vi "实时小时数据处理整合 (子VI).vi"(11 "枚举":enum16{"实时数据排序", "小时数据排序"}(ring)) -> (3 "已排序的数组":string[](array[string]))   [LabVIEW 2016, in "数据传输系统.lvlib"]
uses:
  <userlib>/_OpenG.lib/array/array.llb/Remove Duplicates from 1D Array (String)__ogtk.vi
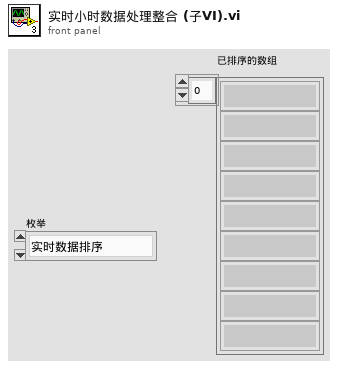
[diagram p1: front panel]
types:
  T1 = cluster{"PH":string[][], "CODCr":string[][], "氨氮":string[][], "CODMn":string[][], "总氮":string[][], "总磷":string[][], "电导率":string[][], "水温":string[][], "DO":string[][], "浊度":string[][], "叶绿素":string[][], "藻密度":string[][], "铜":string[][], "盐度":string[][], "水位":string[][], "流速":string[][], "瞬时流量":string[][], "累积流量":string[][], "亚硝酸盐":string[][], "硫化物":string[][], "ORP":string[][], "铅":string[][], "镉":string[][], "锌":string[][], "镍":string[][], "锰":string[][], "汞":string[][], "气温":string[][], "气压":string[][], "风速":string[][], "风向":string[][], "盐度 2":string[][], "磷酸盐":string[][], "硝氮":string[][], "氟化物":string[][], "挥发酚":string[][], "氯化物":string[][], "蓝绿藻":string[][]}
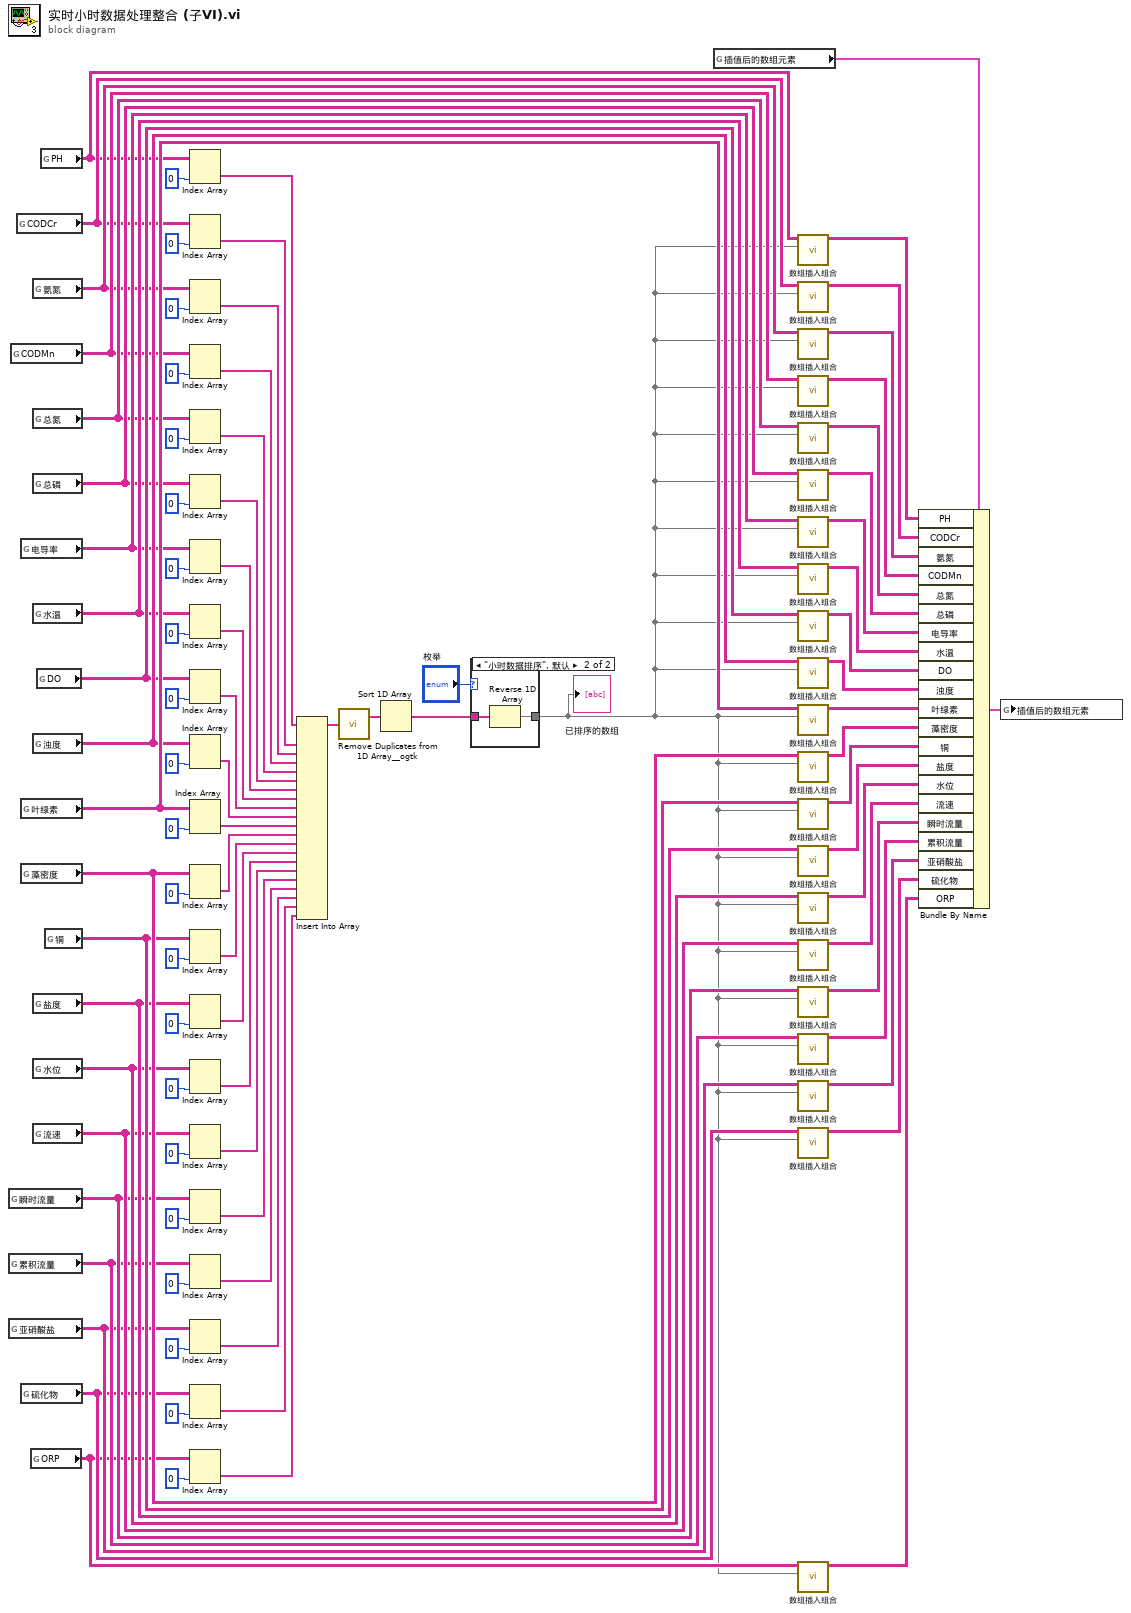
[diagram p0: block diagram]
diagram:
  n1 = global read "全局 所有参数.vi" "瞬时流量"() -> (w23:string[][])
  n2 = global read "全局 所有参数.vi" "累积流量"() -> (w22:string[][])
  n3 = global read "全局 所有参数.vi" "亚硝酸盐"() -> (w13:string[][])
  n4 = global read "全局 所有参数.vi" "CODMn"() -> (w72:string[][])
  n5 = global read "全局 所有参数.vi" "CODCr"() -> (w70:string[][])
  n6 = global read "全局 所有参数.vi" "电导率"() -> (w75:string[][])
  n7 = global read "全局 所有参数.vi" "叶绿素"() -> (w79:string[][])
  n8 = global read "全局 所有参数.vi" "藻密度"() -> (w80:string[][])
  n9 = global read "全局 所有参数.vi" "硫化物"() -> (w10:string[][])
  n10 = global read "全局 所有参数.vi" "ORP"() -> (w9:string[][])
  n11 = global read "全局 所有参数.vi" "氨氮"() -> (w71:string[][])
  n12 = global read "全局 所有参数.vi" "总氮"() -> (w73:string[][])
  n13 = global read "全局 所有参数.vi" "总磷"() -> (w74:string[][])
  n14 = global read "全局 所有参数.vi" "水温"() -> (w76:string[][])
  n15 = global read "全局 所有参数.vi" "浊度"() -> (w78:string[][])
  n16 = global read "全局 所有参数.vi" "盐度"() -> (w38:string[][])
  n17 = global read "全局 所有参数.vi" "水位"() -> (w29:string[][])
  n18 = global read "全局 所有参数.vi" "流速"() -> (w27:string[][])
  n19 = global read "全局 所有参数.vi" "DO"() -> (w77:string[][])
  n20 = global read "全局 所有参数.vi" "PH"() -> (w68:string[][])
  n21 = global read "全局 所有参数.vi" "铜"() -> (w39:string[][])
  n22 = Index Array(array=w68, index (col)=0 ("索引 (行)")) -> (element=w55:string[])  [unwired: 1 in]
  n23 = Index Array(array=w70, index (col)=0 ("索引 (行)")) -> (element=w56:string[])  [unwired: 1 in]
  n24 = Index Array(array=w71, index (col)=0 ("索引 (行)")) -> (element=w57:string[])  [unwired: 1 in]
  n25 = Index Array(array=w72, index (col)=0 ("索引 (行)")) -> (element=w58:string[])  [unwired: 1 in]
  n26 = Index Array(array=w73, index (col)=0 ("索引 (行)")) -> (element=w59:string[])  [unwired: 1 in]
  n27 = Index Array(array=w74, index (col)=0 ("索引 (行)")) -> (element=w60:string[])  [unwired: 1 in]
  n28 = Index Array(array=w75, index (col)=0 ("索引 (行)")) -> (element=w61:string[])  [unwired: 1 in]
  n29 = Index Array(array=w76, index (col)=0 ("索引 (行)")) -> (element=w62:string[])  [unwired: 1 in]
  n30 = Index Array(array=w77, index (col)=0 ("索引 (行)")) -> (element=w63:string[])  [unwired: 1 in]
  n31 = Index Array(array=w78, index (col)=0 ("索引 (行)")) -> (element=w64:string[])  [unwired: 1 in]
  n32 = Index Array(array=w79, index (col)=0 ("索引 (行)")) -> (element=w65:string[])  [unwired: 1 in]
  n33 = Index Array(array=w80, index (col)=0 ("索引 (行)")) -> (element=w66:string[])  [unwired: 1 in]
  n34 = Index Array(array=w39, index (col)=0 ("索引 (行)")) -> (element=w37:string[])  [unwired: 1 in]
  n35 = Index Array(array=w38, index (col)=0 ("索引 (行)")) -> (element=w36:string[])  [unwired: 1 in]
  n36 = Index Array(array=w29, index (col)=0 ("索引 (列)")) -> (element=w30:string[])  [unwired: 1 in]
  n37 = Index Array(array=w27, index (col)=0 ("索引 (列)")) -> (element=w26:string[])  [unwired: 1 in]
  n38 = Index Array(array=w23, index (col)=0 ("索引 (列)")) -> (element=w20:string[])  [unwired: 1 in]
  n39 = Index Array(array=w22, index (col)=0 ("索引 (列)")) -> (element=w21:string[])  [unwired: 1 in]
  n40 = Index Array(array=w13, index (col)=0 ("索引 (列)")) -> (element=w3:string[])  [unwired: 1 in]
  n41 = Index Array(array=w10, index (col)=0 ("索引 (列)")) -> (element=w4:string[])  [unwired: 1 in]
  n42 = Index Array(array=w9, index (col)=0 ("索引 (列)")) -> (element=w5:string[])  [unwired: 1 in]
  n43 = Insert Into Array(array=w55, new element #1=w56, new element #2=w57, new element #3=w58, new element #4=w59, new element #5=w60, new element #6=w61, new element #7=w62, new element #8=w63, new element #9=w64, new element #10=w65, new element #11=w66, new element #12=w37, new element #13=w36, new element #14=w30, new element #15=w26, new element #16=w20, new element #17=w21, new element #18=w3, new element #19=w4, new element #20=w5) -> (w67:string[])  [unwired: 1 in]
  n44 = call-poly <userlib>:"Remove Duplicates from 1D Array__ogtk.vi"("Input Array"=w67) -> ("Output Array"=w54:string[])  [unwired: 1 out]
  n45 = Sort 1D Array(array=w54) -> (sorted array=w40:string[])
  n46 = case shown="\"小时数据排序\", 默认" "枚举" {
    tunnel: w40 -> [w92 w94]
    tunnel: [w92 w93] -> w6
    frame "实时数据排序" {
    }
    frame "小时数据排序", Default {
      n47 = Reverse 1D Array(array=w94) -> (reversed array=w93:string[])
    }
  }
  "已排序的数组" <- w6
  n48 = global read "插值后的新数组.vi" "插值后的数组元素"() -> (w15:T1)
  n49 = call "数组插入组合.vi"("排序后的一维数组"=w6, "输入数组"=w68) -> ("输出结果"=w69:string[][])  [unwired: 9 in]
  n50 = call "数组插入组合.vi"("排序后的一维数组"=w6, "输入数组"=w70) -> ("输出结果"=w81:string[][])  [unwired: 9 in]
  n51 = call "数组插入组合.vi"("排序后的一维数组"=w6, "输入数组"=w71) -> ("输出结果"=w82:string[][])  [unwired: 9 in]
  n52 = call "数组插入组合.vi"("排序后的一维数组"=w6, "输入数组"=w72) -> ("输出结果"=w83:string[][])  [unwired: 9 in]
  n53 = call "数组插入组合.vi"("排序后的一维数组"=w6, "输入数组"=w73) -> ("输出结果"=w84:string[][])  [unwired: 9 in]
  n54 = call "数组插入组合.vi"("排序后的一维数组"=w6, "输入数组"=w74) -> ("输出结果"=w85:string[][])  [unwired: 9 in]
  n55 = call "数组插入组合.vi"("排序后的一维数组"=w6, "输入数组"=w75) -> ("输出结果"=w86:string[][])  [unwired: 9 in]
  n56 = call "数组插入组合.vi"("排序后的一维数组"=w6, "输入数组"=w76) -> ("输出结果"=w87:string[][])  [unwired: 9 in]
  n57 = call "数组插入组合.vi"("排序后的一维数组"=w6, "输入数组"=w77) -> ("输出结果"=w88:string[][])  [unwired: 9 in]
  n58 = call "数组插入组合.vi"("排序后的一维数组"=w6, "输入数组"=w78) -> ("输出结果"=w89:string[][])  [unwired: 9 in]
  n59 = call "数组插入组合.vi"("排序后的一维数组"=w6, "输入数组"=w79) -> ("输出结果"=w90:string[][])  [unwired: 9 in]
  n60 = call "数组插入组合.vi"("排序后的一维数组"=w6, "输入数组"=w80) -> ("输出结果"=w91:string[][])  [unwired: 9 in]
  n61 = call "数组插入组合.vi"("排序后的一维数组"=w6, "输入数组"=w39) -> ("输出结果"=w35:string[][])  [unwired: 9 in]
  n62 = call "数组插入组合.vi"("排序后的一维数组"=w6, "输入数组"=w38) -> ("输出结果"=w34:string[][])  [unwired: 9 in]
  n63 = call "数组插入组合.vi"("排序后的一维数组"=w6, "输入数组"=w29) -> ("输出结果"=w19:string[][])  [unwired: 9 in]
  n64 = call "数组插入组合.vi"("排序后的一维数组"=w6, "输入数组"=w27) -> ("输出结果"=w18:string[][])  [unwired: 9 in]
  n65 = call "数组插入组合.vi"("排序后的一维数组"=w6, "输入数组"=w23) -> ("输出结果"=w17:string[][])  [unwired: 9 in]
  n66 = call "数组插入组合.vi"("排序后的一维数组"=w6, "输入数组"=w22) -> ("输出结果"=w16:string[][])  [unwired: 9 in]
  n67 = call "数组插入组合.vi"("排序后的一维数组"=w6, "输入数组"=w13) -> ("输出结果"=w1:string[][])  [unwired: 9 in]
  n68 = call "数组插入组合.vi"("排序后的一维数组"=w6, "输入数组"=w10) -> ("输出结果"=w2:string[][])  [unwired: 9 in]
  n69 = call "数组插入组合.vi"("排序后的一维数组"=w6, "输入数组"=w9) -> ("输出结果"=w7:string[][])  [unwired: 9 in]
  n70 = Bundle By Name(cluster=w15, "PH"=w69, "CODCr"=w81, "氨氮"=w82, "CODMn"=w83, "总氮"=w84, "总磷"=w85, "电导率"=w86, "水温"=w87, "DO"=w88, "浊度"=w89, "叶绿素"=w90, "藻密度"=w91, "铜"=w35, "盐度"=w34, "水位"=w19, "流速"=w18, "瞬时流量"=w17, "累积流量"=w16, "亚硝酸盐"=w1, "硫化物"=w2, "ORP"=w7) -> (w14:T1)
  n71 = global write "插值后的新数组.vi" "插值后的数组元素"(w14) -> ()
